vi "rp_inline_subvi.vi"(6 "Variant in":variant, 7 "Shift Pressed?":bool, 8 "error in (no error)":errorcluster, 10 "QD Combo Box Ref":refnum<vi>, 11 "QD Launch VI Ref":refnum<vi>) -> (0 "error out":errorcluster, 4 "Variant out":variant)   [LabVIEW 2019]
doc: "Inline the selected SubVI into the current block diagram. Ctrl-Shift wraps the content in a sequence structure.\n\nCreated by: Ryan Pacini\n\nDefault Shortcut - [L]"
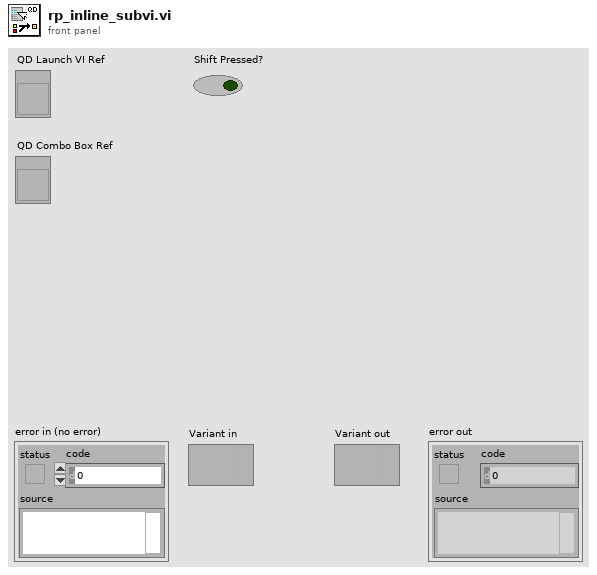
[diagram p1: front panel]
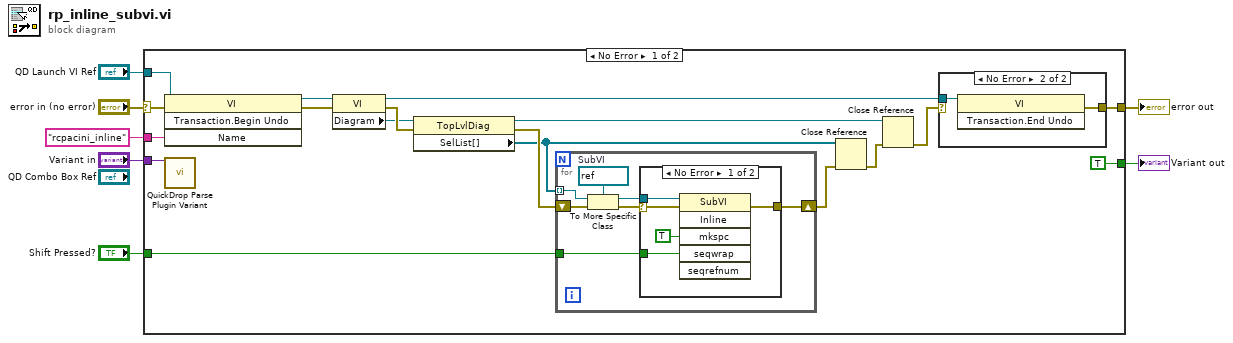
[diagram p0: block diagram]
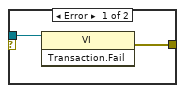
[diagram p3: hidden frame]
diagram:
  n1 = case shown="No Error" "error in (no error)" {
    selector: "error in (no error)" -> [w25 w42]
    tunnel: [w24 w42] -> w3
    tunnel: "QD Launch VI Ref" -> [w21 _]
    tunnel: "rcpacini_inline" ("Undo Name") -> [w23 _]
    tunnel: [TRUE _] -> w4
    tunnel: "Shift Pressed?" -> [w12 _]
    tunnel: "Variant in" -> [w8 _]
    frame No Error {
      n2 = invoke class="VI" method="Transaction.Begin Undo"(reference=w21, error in=w25, "Name"=w23) -> (reference out=w19:refnum<vi>, error out=w20:errorcluster)  [unwired: 1 in, 2 out]
      n3 = call <vilib>:"QuickDrop Parse Plugin Variant.vi"("QDKS Variant in"=w8) -> ()  [unwired: 12 in, 3 out]
      n4 = property class="VI"(reference=w19, error in=w20) -> (reference out=w9:refnum<vi>, error out=w17:errorcluster, "Diagram"=w11:refnum<vi>)
      n5 = property class="TopLvlDiag"(reference=w11, error in=w17) -> (reference out=w10:refnum<vi>, error out=w16:errorcluster, "SelList[]"=w14:refnum<vi>[])
      n6 = for {
        shift-right: [w30] -> w15
        shift-left: w16 -> [w32]
        tunnel: w14 -> [w27] mode=indexing
        tunnel: w12 -> [w26]
        w31 = refnum<vi> refnum  # SubVI
        n7 = To More Specific Class(target class=w31, reference=w27, error in=w32) -> (specific class reference=w29:refnum<vi>, error out=w28:errorcluster)
        n8 = case shown="No Error" w28 {
          selector: w28 -> [w34 _]
          tunnel: [w37 _] -> w30
          tunnel: w29 -> [w35 _]
          tunnel: w26 -> [w33 _]
          frame No Error {
            n9 = invoke class="SubVI" method="Inline"(reference=w35, error in=w34, "mkspc"=TRUE ("Make Space in Block Diagram"), "seqwrap"=w33) -> (error out=w37:errorcluster)  [unwired: 2 in, 5 out]
          }
          frame Error {
          }
        }
      }
      n10 = Close Reference(reference=w14, error in (no error)=w15) -> (error out=w13:errorcluster)
      n11 = Close Reference(reference=w10, error in (no error)=w13) -> (error out=w18:errorcluster)
      n12 = case shown="No Error" w18 {
        tunnel: w9 -> [w38 w40]
        tunnel: [w39 w41] -> w24
        frame Error {
          n13 = invoke class="VI" method="Transaction.Fail"(reference=w38) -> (error out=w39:errorcluster)  [unwired: 2 in, 2 out]
        }
        frame No Error {
          n14 = invoke class="VI" method="Transaction.End Undo"(reference=w40) -> (error out=w41:errorcluster)  [unwired: 2 in, 2 out]
        }
      }
    }
    frame Error {
    }
  }
  "error out" <- w3
  "Variant out" <- w4
